vi "demo_sinanju_hub.vi"() -> ()   [LabVIEW 2017]
panel:
  out "VISA资源名称输出 2":refnum<visa-resource-name>
  out "VISA资源名称输出":refnum<visa-resource-name>
  in  "ip 2":string="192.168.1.44"
  in  "ip":string="127.0.0.1"
  in  "停止":bool
  in  "name 2":string="mrx-t4"
  out "数字 5":i32
  out "数字 4":i32
  out "数字 3":i32
  out "数字 2":i32
  in  "name":string="hub1"
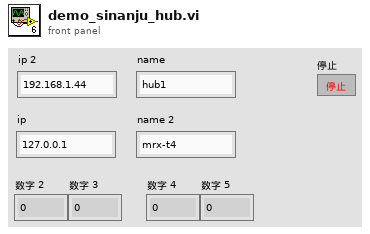
[diagram p1: front panel]
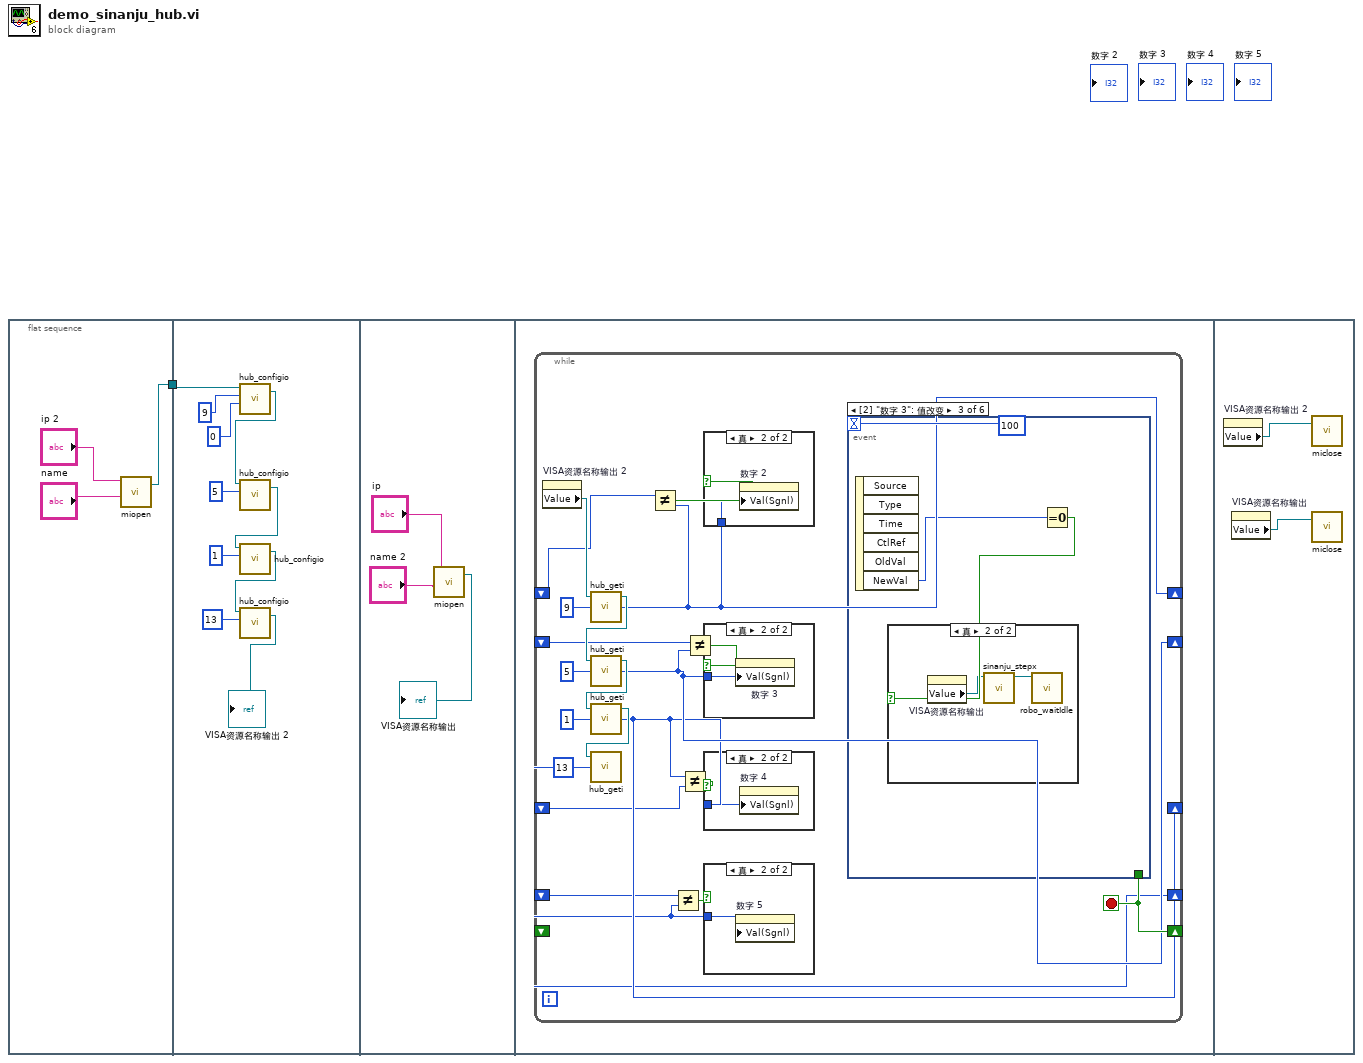
[diagram p0: block diagram]
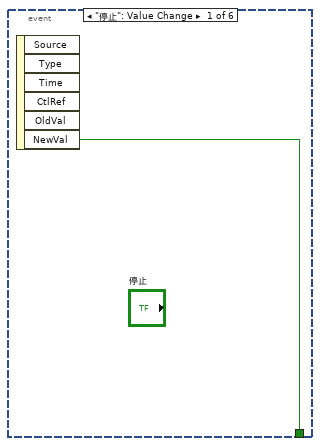
[diagram p6: hidden frame]
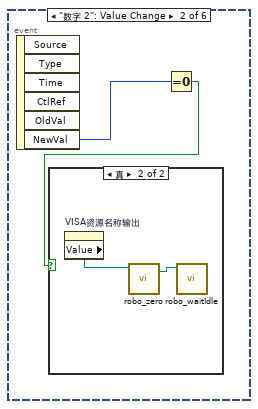
[diagram p7: hidden frame]
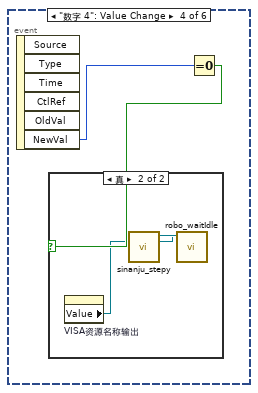
[diagram p10: hidden frame]
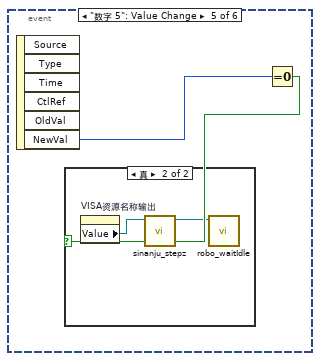
[diagram p12: hidden frame]
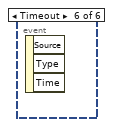
[diagram p14: hidden frame]
diagram:
  n1 = flat-sequence {
    tunnel: [w2] -> w1
    tunnel: w1 -> [w6]
    frame #0 {
      n2 = call "miopen.vi"("name"="name", "ip"="ip 2") -> ("VISA资源名称输出"=w2:refnum<visa-resource-name>)  [unwired: 2 in, 1 out]
    }
    frame #1 {
      n3 = call "hub_configio.vi"("输入 2"=0, "输入 1"=9, "VISA资源名称"=w6) -> ("VISA资源名称输出"=w13:refnum<visa-resource-name>)  [unwired: 1 in, 1 out]
      n4 = call "hub_configio.vi"("输入 1"=5, "VISA资源名称"=w13) -> ("VISA资源名称输出"=w12:refnum<visa-resource-name>)  [unwired: 2 in, 1 out]
      n5 = call "hub_configio.vi"("输入 1"=1, "VISA资源名称"=w12) -> ("VISA资源名称输出"=w11:refnum<visa-resource-name>)  [unwired: 2 in, 1 out]
      n6 = call "hub_configio.vi"("输入 1"=13, "VISA资源名称"=w11) -> ("VISA资源名称输出"=→"VISA资源名称输出 2":refnum<visa-resource-name>)  [unwired: 2 in, 1 out]
    }
    frame #2 {
      n7 = call "miopen.vi"("name"="name 2", "ip"="ip") -> ("VISA资源名称输出"=→"VISA资源名称输出":refnum<visa-resource-name>)  [unwired: 2 in, 1 out]
    }
    frame #3 {
      n8 = while {
        shift-right: [w36] -> _
        shift-left: _ -> [_]
        shift-right: [w28] -> _
        shift-left: _ -> [w29]
        shift-right: [w25] -> _
        shift-left: _ -> [w26]
        shift-right: [w23] -> _
        shift-left: _ -> [w22]
        shift-right: [w20] -> _
        shift-left: _ -> [w21]
        stop <- w36 stop-if-true
        n9 = property on="VISA资源名称输出 2" class="VISAName"() -> ("Value"=w35:refnum<visa-resource-name>)  [unwired: 2 in, 2 out]
        n10 = call "hub_geti.vi"("输入 1"=9, "VISA资源名称"=w35) -> ("数字"=w28:i32, "VISA资源名称输出"=w39:refnum<visa-resource-name>)  [unwired: 1 in, 1 out]
        n11 = call "hub_geti.vi"("输入 1"=5, "VISA资源名称"=w39) -> ("数字"=w25:i32, "VISA资源名称输出"=w38:refnum<visa-resource-name>)  [unwired: 1 in, 1 out]
        n12 = call "hub_geti.vi"("输入 1"=1, "VISA资源名称"=w38) -> ("数字"=w23:i32, "VISA资源名称输出"=w37:refnum<visa-resource-name>)  [unwired: 1 in, 1 out]
        n13 = call "hub_geti.vi"("输入 1"=13, "VISA资源名称"=w37) -> ("数字"=w20:i32)  [unwired: 1 in, 2 out]
        n14 = Not Equal?(x=w29, y=w28) -> (x != y?=w27:bool)
        n15 = Not Equal?(x=w21, y=w20) -> (x != y?=w19:bool)
        n16 = Not Equal?(x=w23, y=w22) -> (x != y?=w18:bool)
        n17 = Not Equal?(x=w26, y=w25) -> (x != y?=w24:bool)
        n18 = case shown="真" w27 {
          tunnel: w28 -> [_ w43]
          frame False {
          }
          frame True {
            n19 = property on="数字 2" class="DigNum (严格)"("Val(Sgnl)"=w43) -> ()  [unwired: 2 in, 2 out]
          }
        }
        n20 = case shown="真" w24 {
          tunnel: w25 -> [_ w42]
          frame False {
          }
          frame True {
            n21 = property on="数字 3" class="DigNum (严格)"("Val(Sgnl)"=w42) -> ()  [unwired: 2 in, 2 out]
          }
        }
        n22 = case shown="真" w18 {
          tunnel: w23 -> [_ w41]
          frame False {
          }
          frame True {
            n23 = property on="数字 4" class="DigNum (严格)"("Val(Sgnl)"=w41) -> ()  [unwired: 2 in, 2 out]
          }
        }
        n24 = case shown="真" w19 {
          tunnel: w20 -> [_ w40]
          frame False {
          }
          frame True {
            n25 = property on="数字 5" class="DigNum (严格)"("Val(Sgnl)"=w40) -> ()  [unwired: 2 in, 2 out]
          }
        }
        n26 = event shown="[2] \"数字 3\": 值改变" {
          selector: _ -> [_ _ _ _ _ _]
          dyn-events: _ -> [_ _ _ _ _ _]
          timeout: 100 -> [_ _ _ _ _ _]
          tunnel: [w44 _ _ _ _ _] -> w36
          event "停止": Value Change {
            n27 = event-data() -> ("NewVal"=w44:bool)  [unwired: 1 in, 5 out]
          }
          event "数字 2": Value Change {
            n28 = event-data() -> ("NewVal"=w46:i32)  [unwired: 1 in, 5 out]
            n29 = Equal To 0?(x=w46) -> (x = 0?=w45:bool)
            n30 = case shown="真" w45 {
              frame False {
              }
              frame True {
                n31 = property on="VISA资源名称输出" class="VISAName"() -> ("Value"=w48:refnum<visa-resource-name>)  [unwired: 2 in, 2 out]
                n32 = call "robo_zero.vi"("VISA资源名称"=w48) -> ("VISA资源名称输出"=w47:refnum<visa-resource-name>)  [unwired: 3 in, 1 out]
                n33 = call "robo_waitIdle.vi"("VISA资源名称"=w47) -> ()  [unwired: 3 in, 3 out]
              }
            }
          }
          event "数字 3": Value Change {
            n34 = event-data() -> ("NewVal"=w50:i32)  [unwired: 1 in, 5 out]
            n35 = Equal To 0?(x=w50) -> (x = 0?=w49:bool)
            n36 = case shown="真" w49 {
              frame False {
              }
              frame True {
                n37 = property on="VISA资源名称输出" class="VISAName"() -> ("Value"=w52:refnum<visa-resource-name>)  [unwired: 2 in, 2 out]
                n38 = call "sinanju_stepx.vi"("VISA资源名称"=w52) -> ("VISA资源名称输出"=w51:refnum<visa-resource-name>)  [unwired: 9 in, 1 out]
                n39 = call "robo_waitIdle.vi"("VISA资源名称"=w51) -> ()  [unwired: 3 in, 3 out]
              }
            }
          }
          event "数字 4": Value Change {
            n40 = event-data() -> ("NewVal"=w53:i32)  [unwired: 1 in, 5 out]
            n41 = Equal To 0?(x=w53) -> (x = 0?=w54:bool)
            n42 = case shown="真" w54 {
              frame False {
              }
              frame True {
                n43 = property on="VISA资源名称输出" class="VISAName"() -> ("Value"=w55:refnum<visa-resource-name>)  [unwired: 2 in, 2 out]
                n44 = call "sinanju_stepy.vi"("VISA资源名称"=w55) -> ("VISA资源名称输出"=w56:refnum<visa-resource-name>)  [unwired: 9 in, 1 out]
                n45 = call "robo_waitIdle.vi"("VISA资源名称"=w56) -> ()  [unwired: 3 in, 3 out]
              }
            }
          }
          event "数字 5": Value Change {
            n46 = event-data() -> ("NewVal"=w57:i32)  [unwired: 1 in, 5 out]
            n47 = Equal To 0?(x=w57) -> (x = 0?=w58:bool)
            n48 = case shown="真" w58 {
              frame False {
              }
              frame True {
                n49 = property on="VISA资源名称输出" class="VISAName"() -> ("Value"=w59:refnum<visa-resource-name>)  [unwired: 2 in, 2 out]
                n50 = call "sinanju_stepz.vi"("VISA资源名称"=w59) -> ("VISA资源名称输出"=w60:refnum<visa-resource-name>)  [unwired: 9 in, 1 out]
                n51 = call "robo_waitIdle.vi"("VISA资源名称"=w60) -> ()  [unwired: 3 in, 3 out]
              }
            }
          }
          event Timeout {
            n52 = event-data() -> ()  [unwired: 1 in, 3 out]
          }
        }
      }
    }
    frame #4 {
      n53 = property on="VISA资源名称输出 2" class="VISAName"() -> ("Value"=w61:refnum<visa-resource-name>)  [unwired: 2 in, 2 out]
      n54 = property on="VISA资源名称输出" class="VISAName"() -> ("Value"=w62:refnum<visa-resource-name>)  [unwired: 2 in, 2 out]
      n55 = call "miclose.vi"("VISA资源名称"=w61) -> ()  [unwired: 1 in, 1 out]
      n56 = call "miclose.vi"("VISA资源名称"=w62) -> ()  [unwired: 1 in, 1 out]
    }
  }
